vi "oa_Extract First Circle Data sub (1 Channel).vi"(6 "index mode":u16(ring) items=["round to nearest", "round to ceiling"], 7 "reset? (True)":bool, 9 "interpolated pulse positions":dbl[](array[numeric]), 10 "speed profile":T1 {"speed [RPM]" format="%.2f"; "time [s]" format="%.2f"}, 11 "resampled signal":cluster{"r0":dbl, "dr":dbl, "Y":dbl[]}) -> (1 "interpolated pulse positions out":dbl[](array[numeric]), 3 "resampled signal out":cluster{"r0":dbl, "dr":dbl, "Y":dbl[]})   [LabVIEW 2017]
uses:
  <vilib>/addons/Sound and Vibration/Order Analysis/Tach Process/SubVIs/speed profile.ctl
  <vilib>/addons/Sound and Vibration/Order Analysis/Tach Process/SoundVib_TachProcess.lvlib
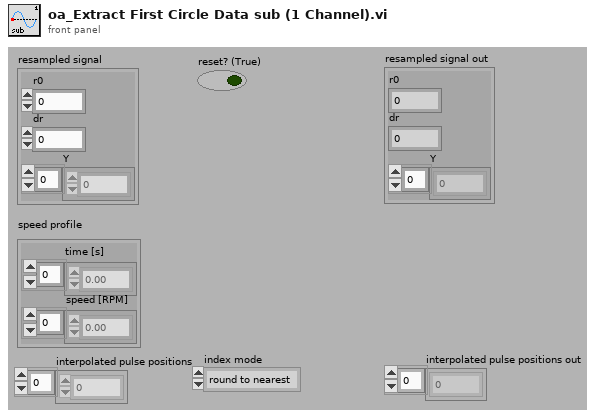
[diagram p1: front panel]
types:
  T1 = typedef "SoundVib_TachProcess.lvlib/speed profile.ctl" = cluster{"time [s]":dbl[], "speed [RPM]":dbl[]}
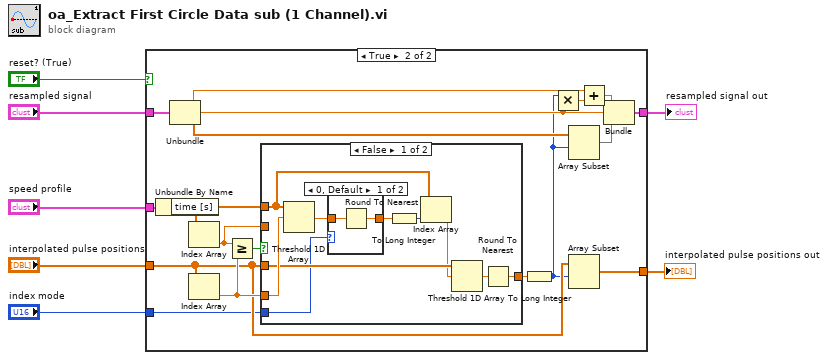
[diagram p0: block diagram]
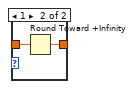
[diagram p3: hidden frame]
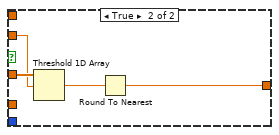
[diagram p4: hidden frame]
diagram:
  n1 = case shown="True" "reset? (True)" {
    tunnel: [w9 w20] -> w4
    tunnel: "speed profile" -> [_ w27]
    tunnel: "interpolated pulse positions" -> [w8 w13]
    tunnel: "resampled signal" -> [w9 w17]
    tunnel: [w8 w11] -> w2
    tunnel: "index mode" -> [_ w10]
    frame False {
    }
    frame True {
      n2 = Unbundle By Name(w27) -> ("time [s]"=w24:dbl[])
      n3 = Unbundle(w17) -> ("r0"=w14:dbl, "dr"=w16:dbl, "Y"=w15:dbl[])
      n4 = Index Array(array=w24) -> (element=w25:dbl)  [unwired: 1 in]
      n5 = Index Array(array=w13) -> (element=w23:dbl)  [unwired: 1 in]
      n6 = Greater Or Equal?(x=w25, y=w23) -> (x >= y?=w26:bool)
      n7 = case shown="False" w26 {
        tunnel: w25 -> [_ w44]
        tunnel: w13 -> [w32 w45]
        tunnel: [w29 w42] -> w22
        tunnel: w24 -> [w34 _]
        tunnel: w23 -> [w37 _]
        tunnel: w10 -> [w28 _]
        frame False {
          n8 = Threshold 1D Array(2:w37, 3:w34) -> (0:w36:dbl)  [unwired: 1 in]
          n9 = case shown="0, Default" w28 {
            tunnel: w36 -> [w38 w41]
            tunnel: [w39 w40] -> w35
            frame 0, Default {
              n10 = Round To Nearest(number=w38) -> (nearest integer value=w39:dbl)
            }
            frame 1 {
              n11 = Round Toward +Infinity(x=w41) -> (ceil(x): smallest int >= x=w40:dbl)
            }
          }
          n12 = To Long Integer(number=w35) -> (32bit integer=w33:i32)
          n13 = Index Array(array=w34, index=w33) -> (element=w31:dbl)
          n14 = Threshold 1D Array(2:w31, 3:w32) -> (0:w30:dbl)  [unwired: 1 in]
          n15 = Round To Nearest(number=w30) -> (nearest integer value=w29:dbl)
        }
        frame True {
          n16 = Threshold 1D Array(2:w44, 3:w45) -> (0:w43:dbl)  [unwired: 1 in]
          n17 = Round To Nearest(number=w43) -> (nearest integer value=w42:dbl)
        }
      }
      n18 = To Long Integer(number=w22) -> (32bit integer=w12:i32)
      n19 = Multiply(x=w12, y=w16) -> (x*y=w19:dbl)
      n20 = Array Subset(array=w15, index=w12) -> (w21:dbl[])  [unwired: 1 in]
      n21 = Array Subset(array=w13, index=w12) -> (w11:dbl[])  [unwired: 1 in]
      n22 = Add(x=w14, y=w19) -> (x+y=w18:dbl)
      n23 = Bundle(w18, "dr"=w16, w21) -> (w20:cluster{dbl, "dr":dbl, dbl[]})  [unwired: 1 in]
    }
  }
  "resampled signal out" <- w4
  "interpolated pulse positions out" <- w2
